vi "Find co-incident points wtf.vi"(8 "Half of the number of integers to search":i32=25, 9 "Co-incidence Tolerance":dbl=0.05, 10 "Mutual Viewing Angle":dbl[](array[numeric])=[0.0, 1.0, 0.0], 11 "Grain Boundary Macro Definition":T2={"Grain 1 Orientation"=[1.0, 0.0, 0.0], "Grain 2 Orientation"=[1.0, 1.0, 0.0], "Twist Angle (Deg)"=0.0}) -> (3 "Coincident points":dbl[][](array[numeric]))   [LabVIEW 2010]
uses:
  <vilib>/Analysis/Matrix/Datatypes/RealMatrix.ctl
  <vilib>/Analysis/Matrix/Numeric/Subtract/Subtract - RM,RM.vi
  <vilib>/Analysis/baseanly.llb/Real Inverse Matrix.vi
  <vilib>/Analysis/baseanly.llb/Real A x B.vi
  <vilib>/Analysis/baseanly.llb/A x Vector.vi
  <vilib>/Analysis/NI_AALPro.lvlib
  <vilib>/Analysis/NI_AALBase.lvlib
  <vilib>/Analysis/Matrix/NI_Matrix.lvlib
panel:
  out "Grain B":T1=[[0.0, 1.0, 0.0], [0.0, 0.0, -1.0], [1.0, 0.0, 0.0]]
  in  "Sort by Cols":i32[](array[numeric])=[0, 1, 2]
  out "Misorientation Matrix":T1=[[0.0, 1.0, 0.0], [0.0, 0.0, -1.0], [1.0, 0.0, 0.0]]
  out "Total Time (ms)":u32
  in  "Lattice vector c":dbl[](array[numeric])=[3.3046962263585, 3.3046962263585, 0.0]
  in  "Lattice vector b":dbl[](array[numeric])=[3.3046962263585, 0.0, 3.3046962263585]
  in  "Lattice vector a":dbl[](array[numeric])=[0.0, 3.3046962263585, 3.3046962263585]
  out "Change of Basis Matrix":T1=[[0.15129983688423865, -0.15129983688423865, -0.15129983688423865], [-0.15129983688423865, -0.15129983688423865, 0.15129983688423865], [0.15129983688423865, 0.15129983688423865, 0.15129983688423865]]
  out "Grain A":T1=[[0.0, 1.0, 0.0], [0.0, 0.0, -1.0], [1.0, 0.0, 0.0]]
  # "Sort by distance from GB plane and then by near-coincidence."
  # "Primitives"
  # "Grain 1 Lattice"
  # "Co-incident radius"
  # "Distance from GB"
  # "Real space1 x,y,z"
  # "Lattice 1 a,b,c"
  # "Difference Vector a,b,c, |r-r'|"
  # "Distance from zero"
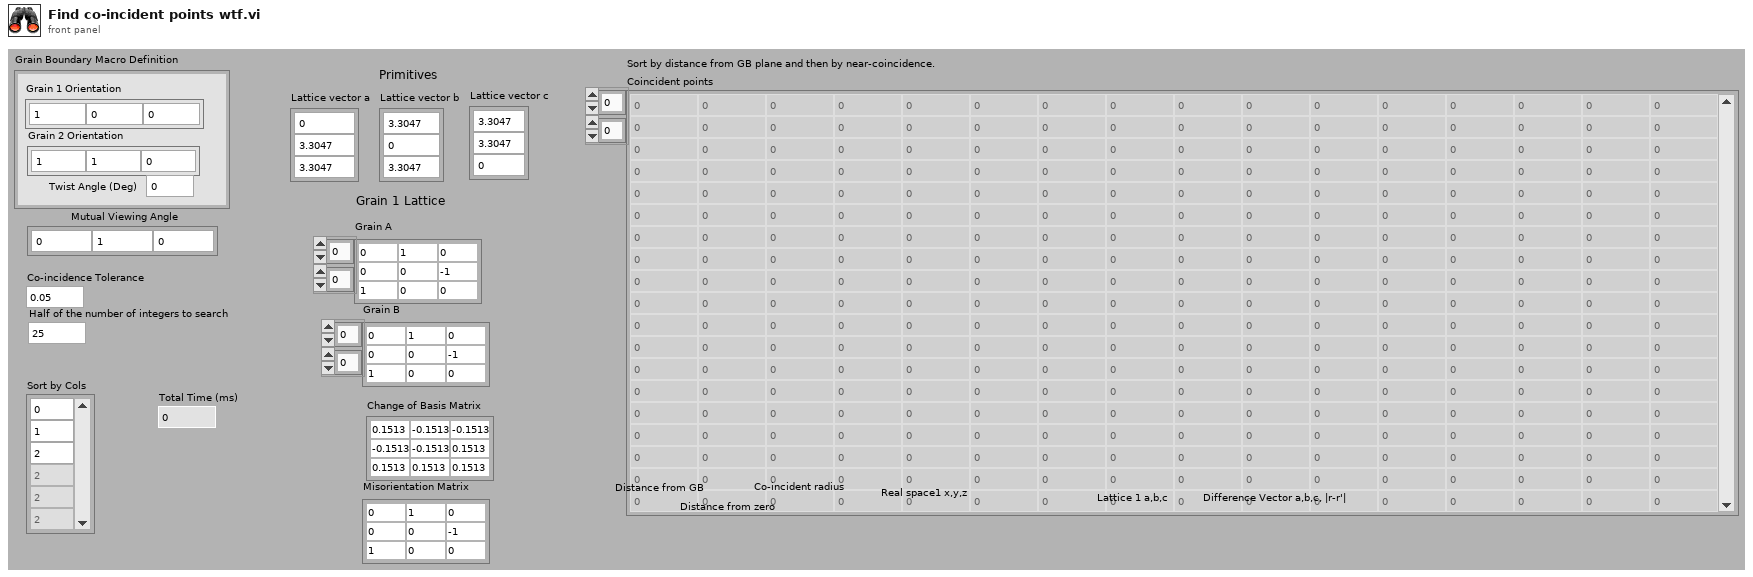
[diagram p1: front panel]
types:
  T1 = typedef "NI_Matrix.lvlib/RealMatrix.ctl" = dbl[][]
  T2 = cluster{"Grain 1 Orientation":dbl[], "Grain 2 Orientation":dbl[], "Twist Angle (Deg)":dbl}
  T3 = cluster{"Grain 1 Orientation":dbl[], "Grain 2 Orientation":dbl[], "Twist Angle (Deg)":dbl, "Mutual Viewing Angle 2":dbl[]}
  T4 = cluster{"Misorientation Angle":dbl, "Misorientation Axis, o":dbl[], "Misorientation Matrix":T1}
  T5 = cluster{"[0]":dbl, "[1]":dbl, "[2]":dbl, "[3]":dbl, "[4]":dbl, "[5]":dbl, "[6]":dbl, "[7]":dbl, "[8]":dbl, "[9]":dbl, "[10]":dbl, "[11]":dbl, "[12]":dbl, "[13]":dbl, "[14]":dbl}
  T6 = cluster{"[0]":dbl, "[1]":dbl, "[2]":dbl, "[3]":dbl, "[4]":dbl, "[5]":dbl, "[6]":dbl, "[7]":dbl, "[8]":dbl, "[9]":dbl, "[10]":dbl, "[11]":dbl, "[12]":dbl, "[13]":dbl, "[14]":dbl}[]
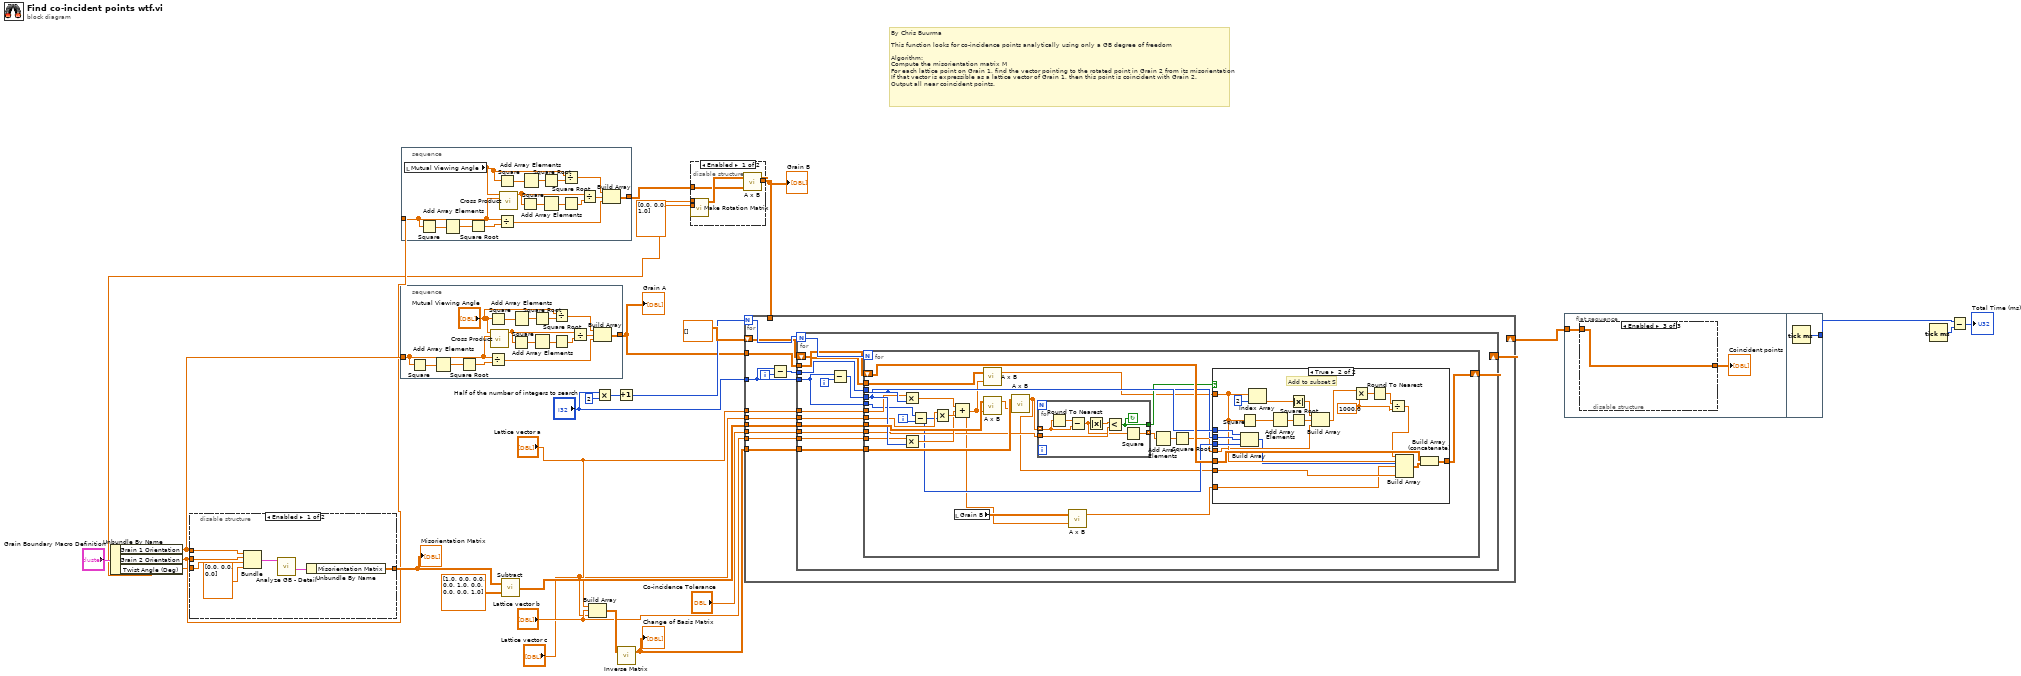
[diagram p0: block diagram]
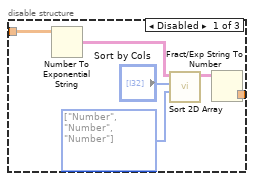
[diagram p3: hidden frame]
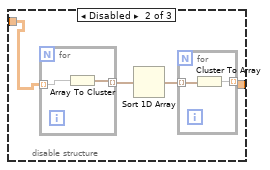
[diagram p4: hidden frame]
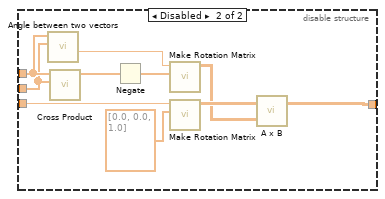
[diagram p5: hidden frame]
diagram:
  # "By Chris Buurma\n\nThis function looks for co-incidence points analytically using only a GB degree of freedom\n\nAlgorithm:\nCompute the misorientation matrix M\nFor each lattice point on Grain 1, find the vector pointing to the rotated point in Grain 2 from its misorientation\nIf that vector is expressible as a lattice vector of Grain 1, then this point is coincident with Grain 2.\nOutput all near coincident points."
  n1 = Unbundle By Name("Grain Boundary Macro Definition") -> ("Grain 1 Orientation"=w10:dbl[], "Grain 2 Orientation"=w5:dbl[], "Twist Angle (Deg)"=w4:dbl)
  n2 = disable-structure shown="Enabled" {
    disable-tunnel: w10 -> [w33 w36]
    disable-tunnel: w5 -> [w32 w35]
    disable-tunnel: w4 -> [w31 w41]
    disable-tunnel: [w27 w39] -> w15
    frame Enabled {
      n3 = Bundle("Grain 1 Orientation"=w33, "Grain 2 Orientation"=w32, "Twist Angle (Deg)"=w31, "Mutual Viewing Angle 2"=dbl[] [0.0, 0.0, 0.0]) -> (w29:T3)  [unwired: 1 in]
      n4 = call "Analyze GB - Detail.vi"("Grain Boundary Definition"=w29) -> ("Misorientation"=w28:T4)  [unwired: 3 in, 7 out]
      n5 = Unbundle By Name(w28) -> ("Misorientation Matrix"=w27:T1)
    }
    frame Disabled {
      n6 = call "Angle between two vectors.vi"("Vector 2"=w35, "Vector 1"=w36) -> ("Angle (Degrees)"=w34:dbl)  [unwired: 7 in, 2 out]
      n7 = call <vilib>:"Cross Product.vi"("B Vector"=w35, "A Vector"=w36) -> ("Cross Product"=w43:dbl[])  [unwired: 8 in, 1 out]
      n8 = Negate(x=w43) -> (-x=w37:dbl[])
      n9 = call "Make Rotation Matrix.vi"("Rotation Axis"=w37, "Rotation Angle (Degree)"=w34) -> ("Rotation Matrix"=w38:T1)  [unwired: 9 in]
      n10 = call "Make Rotation Matrix.vi"("Rotation Axis"=dbl[] [0.0, 0.0, 1.0], "Rotation Angle (Degree)"=w41) -> ("Rotation Matrix"=w40:T1)  [unwired: 9 in]
      n11 = call-poly <vilib>:"A x B.vi"("B"=w38, "A"=w40) -> ("A x B"=w39:T1)  [unwired: 1 out]
    }
  }
  "Misorientation Matrix" <- w15
  n12 = stacked-sequence {
    tunnel: [w46] -> w6
    tunnel: w10 -> [w44]
    frame #0 {
      n13 = Square(x=w44) -> (x^2=w57:dbl[])
      n14 = Add Array Elements(numeric array=w57) -> (sum=w56:dbl)
      n15 = Square Root(x=w56) -> (sqrt(x)=w55:dbl)
      n16 = Square(x="Mutual Viewing Angle") -> (x^2=w53:dbl[])
      n17 = Divide(x=w44, y=w55) -> (x/y=w59:dbl[])
      n18 = call <vilib>:"Cross Product.vi"("B Vector"=w44, "A Vector"="Mutual Viewing Angle") -> ("Cross Product"=w48:dbl[])  [unwired: 8 in, 1 out]
      n19 = Square(x=w48) -> (x^2=w50:dbl[])
      n20 = Add Array Elements(numeric array=w53) -> (sum=w54:dbl)
      n21 = Square Root(x=w54) -> (sqrt(x)=w51:dbl)
      n22 = Add Array Elements(numeric array=w50) -> (sum=w49:dbl)
      n23 = Divide(x="Mutual Viewing Angle", y=w51) -> (x/y=w52:dbl[])
      n24 = Square Root(x=w49) -> (sqrt(x)=w47:dbl)
      n25 = Divide(x=w48, y=w47) -> (x/y=w58:dbl[])
      n26 = Build Array(w52, w58, w59) -> (w46:T1)
    }
  }
  "Grain A" <- w6
  n27 = stacked-sequence {
    tunnel: [w62] -> w1
    tunnel: w5 -> [w60]
    frame #0 {
      n28 = local read "Mutual Viewing Angle"() -> (w61:dbl[])
      n29 = Square(x=w60) -> (x^2=w73:dbl[])
      n30 = Add Array Elements(numeric array=w73) -> (sum=w72:dbl)
      n31 = Square Root(x=w72) -> (sqrt(x)=w71:dbl)
      n32 = Square(x=w61) -> (x^2=w69:dbl[])
      n33 = Divide(x=w60, y=w71) -> (x/y=w75:dbl[])
      n34 = call <vilib>:"Cross Product.vi"("B Vector"=w60, "A Vector"=w61) -> ("Cross Product"=w64:dbl[])  [unwired: 8 in, 1 out]
      n35 = Square(x=w64) -> (x^2=w66:dbl[])
      n36 = Add Array Elements(numeric array=w69) -> (sum=w70:dbl)
      n37 = Square Root(x=w70) -> (sqrt(x)=w67:dbl)
      n38 = Add Array Elements(numeric array=w66) -> (sum=w65:dbl)
      n39 = Divide(x=w61, y=w67) -> (x/y=w68:dbl[])
      n40 = Square Root(x=w65) -> (sqrt(x)=w63:dbl)
      n41 = Divide(x=w64, y=w63) -> (x/y=w74:dbl[])
      n42 = Build Array(w68, w74, w75) -> (w62:T1)
    }
  }
  n43 = call-poly <vilib>:"Subtract.vi"("Real Matrix B"=T1 [[1.0, 0.0, 0.0], [0.0, 1.0, 0.0], [0.0, 0.0, 1.0]] ("Misorientation Matrix"), "Real Matrix A"=w15) -> ("A - B"=w24:T1)
  n44 = Build Array("Lattice vector a", "Lattice vector b", "Lattice vector c") -> (w19:T1)
  n45 = Multiply(x="Half of the number of integers to search", y=2) -> (x*y=w12:i32)
  n46 = Increment(x=w12) -> (x+1=w11:i32)
  n47 = call-poly <vilib>:"Inverse Matrix.vi"("Input Matrix"=w19) -> ("Inverse Matrix"=w21:T1)  [unwired: 1 in, 1 out]
  "Change of Basis Matrix" <- w21
  n48 = disable-structure shown="Enabled" {
    disable-tunnel: dbl[] [0.0, 0.0, 1.0] ("Rotation Axis") -> [w80 _]
    disable-tunnel: w4 -> [w79 _]
    disable-tunnel: w1 -> [w77 w81]
    disable-tunnel: [w76 w81] -> w3
    frame Enabled {
      n49 = call "Make Rotation Matrix.vi"("Rotation Axis"=w80, "Rotation Angle (Degree)"=w79) -> ("Rotation Matrix"=w78:T1)  [unwired: 9 in]
      n50 = call-poly <vilib>:"A x B.vi"("B"=w77, "A"=w78) -> ("A x B"=w76:T1)  [unwired: 1 out]
    }
    frame Disabled {
    }
  }
  "Grain B" <- w3
  n51 = for {
    N: w11 -> [w93]
    tunnel: w24 -> [w94]
    shift-right: [w92] -> w22
    shift-left: dbl[][] [] -> [w91]
    tunnel: w21 -> [w90]
    tunnel: "Co-incidence Tolerance" -> [w89]
    tunnel: "Lattice vector a" -> [w88]
    tunnel: "Lattice vector b" -> [w87]
    tunnel: "Lattice vector c" -> [w86]
    tunnel: "Half of the number of integers to search" -> [w83]
    tunnel: w6 -> [w82]
    tunnel: w3 -> [_]
    i -> [w85]
    n52 = Subtract(x=w83, y=w85) -> (x-y=w84:i32)
    n53 = for {
      N: w93 -> [w106]
      tunnel: w94 -> [w108]
      tunnel: w84 -> [w107]
      shift-right: [w105] -> w92
      shift-left: w91 -> [w104]
      tunnel: w90 -> [w103]
      tunnel: w89 -> [w102]
      tunnel: w88 -> [w101]
      tunnel: w87 -> [w100]
      tunnel: w86 -> [w99]
      tunnel: w83 -> [w96]
      tunnel: w82 -> [w95]
      i -> [w98]
      n54 = Subtract(x=w96, y=w98) -> (x-y=w97:i32)
      n55 = for {
        N: w106 -> [_]
        tunnel: w108 -> [w134]
        tunnel: w107 -> [w129]
        tunnel: w97 -> [w128]
        shift-right: [w131] -> w105
        shift-left: w104 -> [w130]
        tunnel: w103 -> [w127]
        tunnel: w102 -> [w126]
        tunnel: w101 -> [w124]
        tunnel: w100 -> [w123]
        tunnel: w99 -> [w122]
        tunnel: w96 -> [w120]
        tunnel: w95 -> [w118]
        i -> [w121]
        n56 = Multiply(x=w124, y=w129) -> (x*y=w135:dbl[])
        n57 = Multiply(x=w123, y=w128) -> (x*y=w132:dbl[])
        n58 = Subtract(x=w120, y=w121) -> (x-y=w119:i32)
        n59 = Multiply(x=w122, y=w119) -> (x*y=w133:dbl[])
        n60 = local read "Grain B"() -> (w110:T1)
        n61 = Compound Arithmetic op=ADD(w135, w132, w133) -> (w109:dbl[])
        n62 = call-poly <vilib>:"A x B.vi"("Vector"=w109, "A"=w118) -> ("A x Vector"=w117:dbl[])  [unwired: 1 out]
        n63 = call-poly <vilib>:"A x B.vi"("Vector"=w109, "A"=w134) -> ("A x Vector"=w111:dbl[])  [unwired: 1 out]
        n64 = call-poly <vilib>:"A x B.vi"("Vector"=w111, "A"=w127) -> ("A x Vector"=w112:dbl[])  [unwired: 1 out]
        n65 = for {
          tunnel: w112 -> [w164] mode=indexing
          tunnel: w126 -> [w162]
          tunnel: [w161] -> w125
          tunnel: [w159] -> w116 mode=indexing
          stop <- w161 continue-if-true
          n66 = Round To Nearest(number=w164) -> (nearest integer value=w165:dbl)
          n67 = Subtract(x=w165, y=w164) -> (x-y=w160:dbl)
          n68 = Absolute Value(x=w160) -> (abs(x)=w163:dbl)
          n69 = Less?(x=w163, y=w162) -> (x < y?=w161:bool)
          n70 = Square(x=w160) -> (x^2=w159:dbl)
        }
        n71 = call-poly <vilib>:"A x B.vi"("Vector"=w109, "A"=w110) -> ("A x Vector"=w113:dbl[])  [unwired: 1 out]
        n72 = Add Array Elements(numeric array=w116) -> (sum=w115:dbl)
        n73 = Square Root(x=w115) -> (sqrt(x)=w114:dbl)
        n74 = case shown="True" w125 {
          tunnel: [w136 w158] -> w131
          tunnel: w130 -> [w136 w157]
          tunnel: w129 -> [_ w156]
          tunnel: w128 -> [_ w155]
          tunnel: w119 -> [_ w154]
          tunnel: w112 -> [_ w152]
          tunnel: w117 -> [_ w149]
          tunnel: w114 -> [_ w146]
          tunnel: w113 -> [_ w137]
          frame False {
            # "Do not add"
          }
          frame True {
            w140 = 1000.0 ("y")
            # "Add to subset S"
            n75 = Build Array(w156, w155, w154) -> (w138:i32[])
            n76 = Square(x=w149) -> (x^2=w150:dbl[])
            n77 = Index Array(array=w149, index=2) -> (element=w147:dbl)
            n78 = Add Array Elements(numeric array=w150) -> (sum=w151:dbl)
            n79 = Absolute Value(x=w147) -> (abs(x)=w144:dbl)
            n80 = Square Root(x=w151) -> (sqrt(x)=w145:dbl)
            n81 = Build Array(w144, w145, w146) -> (w141:dbl[])
            n82 = Multiply(x=w141, y=w140) -> (x*y=w142:dbl[])
            n83 = Round To Nearest(number=w142) -> (nearest integer value=w143:dbl[])
            n84 = Divide(x=w143, y=w140) -> (x/y=w139:dbl[])
            n85 = Build Array(w139, w149, w137, w138, w152) -> (w153:dbl[][])
            n86 = Build Array (concatenate)(w157, w153) -> (w158:dbl[][])
          }
        }
      }
    }
  }
  n87 = flat-sequence {
    tunnel: w22 -> [w167]
    tunnel: [w183] -> w18
    frame #0 {
      n88 = disable-structure shown="Enabled" {
        disable-tunnel: w167 -> [w171 w177 w182]
        disable-tunnel: [w168 w174 w182] -> w166
        frame Disabled {
          w172 = enum16{"String", "Number", "Date-Time"}[] [enum."Number", enum."Number", enum."Number"] items=["String", "Number", "Date-Time"] ("Sort by Datatype Array")
          n89 = Number To Exponential String(number=w171) -> (E-format string=w170:string[][])  [unwired: 3 in]
          n90 = call "Sort 2D Array.vi"("Sort by Datatype Array"=w172, "Sort by Cols"="Sort by Cols", "Input Array"=w170) -> ("Output Array"=w169:string[][])  [unwired: 8 in]
          n91 = Fract/Exp String To Number(string=w169) -> (number=w168:dbl[][])  [unwired: 3 in, 1 out]
        }
        frame Disabled {
          n92 = for {
            tunnel: w177 -> [w181] mode=indexing
            tunnel: [w180] -> w176 mode=indexing
            n93 = Array To Cluster(array=w181) -> (cluster=w180:T5)
          }
          n94 = Sort 1D Array(array=w176) -> (sorted array=w175:T6)
          n95 = for {
            tunnel: w175 -> [w179] mode=indexing
            tunnel: [w178] -> w174 mode=indexing
            n96 = Cluster To Array(cluster=w179) -> (array=w178:dbl[])
          }
        }
        frame Enabled {
        }
      }
      "Coincident points" <- w166
    }
    frame #1 {
      n97 = Tick Count (ms)() -> (millisecond timer value=w183:u32)
    }
  }
  n98 = Tick Count (ms)() -> (millisecond timer value=w17:u32)
  n99 = Subtract(x=w18, y=w17) -> (x-y=→"Total Time (ms)":u32)
